vi "01 LinkTest.vi"(8 "error in (no error)":errorcluster caption="错误输入（无错误）", 9 "超时毫秒":i32=500, 10 "服务端识别":cluster{"本机IP":string, "本机端口":u16}, 11 "TCPServerClass 输入":refnum<class "TCPServerClass.lvclass">) -> (0 "error out":errorcluster caption="错误输出", 2 "成功？":bool, 3 "TCPServerClass 输出":refnum<class "TCPServerClass.lvclass">)   [LabVIEW 2019, in "TCPServerClass.lvclass"]
uses:
  TCPServerClass.lvclass
  TCPServerClass.lvclass/TCPServerClass.ctl
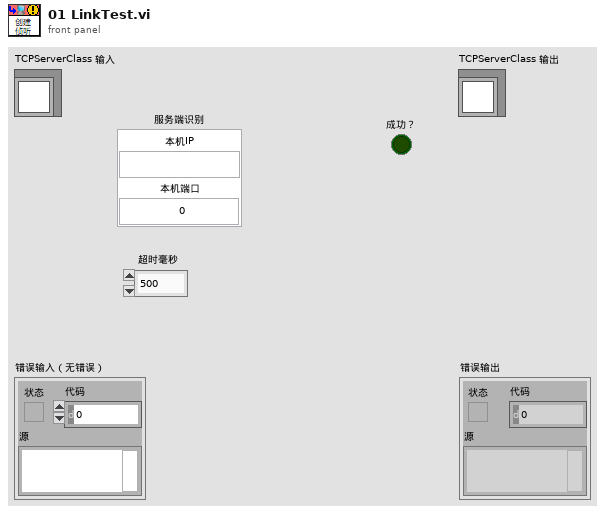
[diagram p1: front panel]
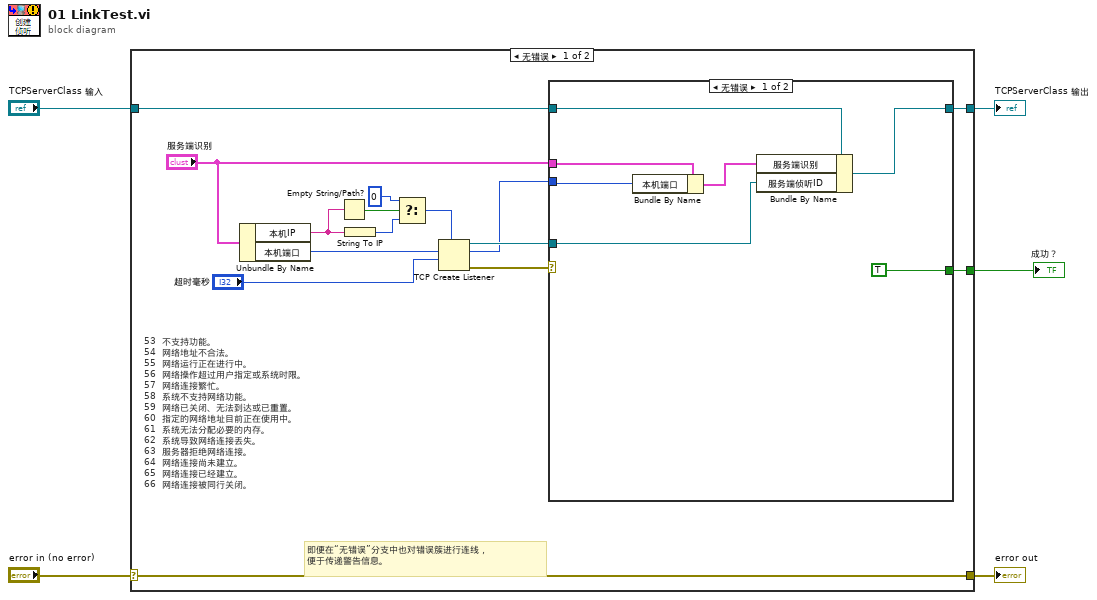
[diagram p0: block diagram]
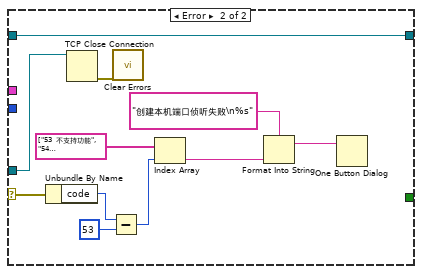
[diagram p2: hidden frame]
diagram:
  n1 = case shown="无错误" "error in (no error)" {
    selector: "error in (no error)" -> [w20 w40]
    tunnel: [w20 w40] -> w4
    tunnel: [w10 w39] -> w2
    tunnel: "TCPServerClass 输入" -> [w11 w39]
    tunnel: [w6 _] -> w1
    frame No Error {
      # "53  不支持功能。\n54  网络地址不合法。\n55  网络运行正在进行中。\n56  网络操作超过用户指定或系统时限。\n57  网络连接繁忙。\n58  系统不支持网络功能。\n59  网络已关闭、无法到达或已重置。\n60  指定的网络地址目前正在使用中。\n61  系统无法分配必要的内存。\n62  系统导致网络连接丢失。\n63  服务器拒绝网络连接。\n64  网络连接尚未建立。\n65  网络连接已经建立。\n66  网络连接被同行关闭。"
      # "即便在“无错误”分支中也对错误簇进行连线，\n便于传递警告信息。"
      n2 = Unbundle By Name("服务端识别") -> ("本机IP"=w13:string, "本机端口"=w14:u16)
      n3 = Empty String/Path?(string/path=w13) -> (empty?=w19:bool)
      n4 = String To IP(1:w13) -> (0:w18:u32)
      n5 = Select(t=u32 0, s=w19, f=w18) -> (s? t:f=w16:u32)
      n6 = TCP Create Listener(7:w16, 9:"超时毫秒", 10:w14) -> (0:w12:errorcluster, 2:w7:u16, 3:w8:refnum<k5>)  [unwired: 2 in]
      n7 = case shown="无错误" w12 {
        selector: w12 -> [_ w36]
        tunnel: w11 -> [w27 w30]
        tunnel: [w26 w30] -> w10
        tunnel: "服务端识别" -> [w24 _]
        tunnel: w8 -> [w25 w29]
        tunnel: w7 -> [w23 _]
        tunnel: [TRUE _] -> w6
        frame No Error {
          n8 = Bundle By Name(cluster=w24, "本机端口"=w23) -> (w22:cluster{"本机IP":string, "本机端口":u16})
          n9 = Bundle By Name(cluster=w27, "服务端识别"=w22, "服务端侦听ID"=w25) -> (w26:refnum<class "TCPServerClass.lvclass">)
        }
        frame Error {
          n10 = Unbundle By Name(w36) -> ("code"=w38:i32)
          n11 = TCP Close Connection(connection ID=w29) -> (error out=w28:errorcluster)  [unwired: 2 in, 1 out]
          n12 = Subtract(x=w38, y=53) -> (x-y=w34:i32)
          n13 = call <vilib>:"Clear Errors.vi"("error in (no error)"=w28) -> ()  [unwired: 5 in, 2 out]
          n14 = Index Array(array=string[] ["53  不支持功能", "54  网络地址不合法", "55  网络运行正在进行中", "56  网络操作超过用户指定或系统时限", "57  网络连接繁忙", "58  系统不支持网络功能", "59  网络已关闭、无法到达或已重置", "60  指定的网络地址目前正在使用中", "61  系统无法分配必要的内存", "62  系统导致网络连接丢失", "63  服务器拒绝网络连接", "64  网络连接尚未建立", "65  网络连接已经建立", "66  网络连接被同行关闭"], index=w34) -> (element=w32:string)
          n15 = Format Into String(format string="创建本机端口侦听失败\n%s" ("格式字符串"), w32) -> (resulting string=w31:string)  [unwired: 2 in, 1 out]
          n16 = One Button Dialog(message=w31) -> ()  [unwired: 1 in, 1 out]
        }
      }
    }
    frame Error {
    }
  }
  "error out" <- w4
  "TCPServerClass 输出" <- w2
  "成功？" <- w1
